vi "Get Relay Position.vi"(8 "error in (no error)":errorcluster, 10 "relay name":string, 11 "SLSC Switch in":refnum<class "SLSC Switch.lvclass">) -> (0 "error out":errorcluster, 2 "position":T1=10 items=["Open"=10, "Closed"=11], 3 "SLSC Switch out":refnum<class "SLSC Switch.lvclass">)   [LabVIEW 2015, in "SLSC Switch.lvclass"]
doc: "Returns the relay position for the relay specified in relay name."
uses:
  SLSC Switch.lvclass
  slscsl/RelayPosition.ctl
  SLSC Switch.lvclass/SLSC Switch.ctl
  Relay Interface/RelayInterface.lvclass
  slscsl/slscsl.lvclass
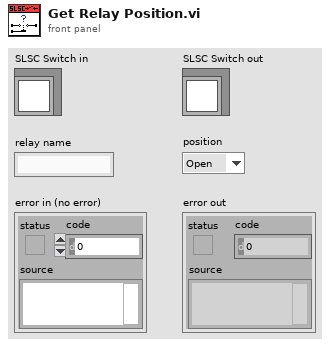
[diagram p1: front panel]
types:
  T1 = typedef "slscsl.lvclass/RelayPosition.ctl" = i32
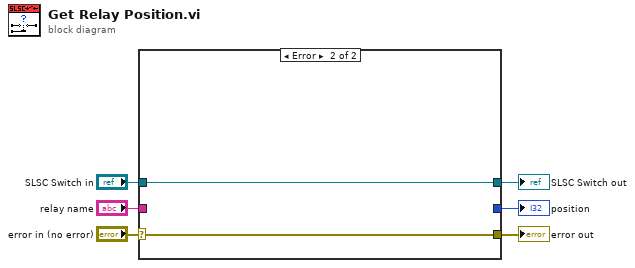
[diagram p0: block diagram]
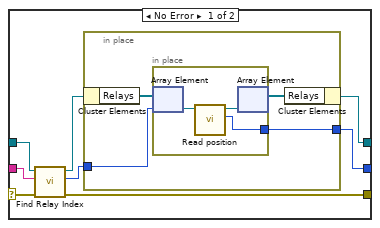
[diagram p2: hidden frame]
diagram:
  n1 = case shown="Error" "error in (no error)" {
    selector: "error in (no error)" -> [w13 w23]
    tunnel: [w11 w23] -> w5
    tunnel: "relay name" -> [w14 _]
    tunnel: [w12 _] -> w3
    tunnel: "SLSC Switch in" -> [w10 w22]
    tunnel: [w9 w22] -> w1
    frame No Error {
      n2 = call "Find Relay Index.vi"("error in (no error)"=w13, "relay string"=w14, "SLSC Switch in"=w10) -> ("error out"=w11:errorcluster, "index"=w8:i32, "SLSC Switch out"=w7:refnum<class "SLSC Switch.lvclass">)  [unwired: 6 in]
      n3 = in-place {
        in-place-border: [w18] -> w12
        in-place-border: w8 -> [w17]
        n4 = in-place-cluster #1(w7) -> ("Relays"=w16:refnum<class "RelayInterface.lvclass">[])
        n5 = in-place {
          in-place-border: [w19] -> w18
          n6 = in-place-array #2(w16, w17) -> (w21:refnum<class "RelayInterface.lvclass">)
          n7 = call-dynamic "Read position.vi"("RelayInterface in"=w21) -> ("position"=w19:T1, "RelayInterface out"=w20:refnum<class "RelayInterface.lvclass">)  [unwired: 9 in]
          n8 = in-place-array #2(w20) -> (w15:refnum<class "RelayInterface.lvclass">[])  [unwired: 1 out]
        }
        n9 = in-place-cluster #1("Relays"=w15) -> (w9:refnum<class "SLSC Switch.lvclass">)
      }
    }
    frame Error {
    }
  }
  "error out" <- w5
  "position" <- w3
  "SLSC Switch out" <- w1
